vi "Test Indeterminate Progress Bar.vi"() -> ()   [LabVIEW 2020]
panel:
  out "Slide 2":cluster{dbl, dbl}(slide) caption="Running script" scale=0.0..100.0
  out "Slide":cluster{dbl, dbl}(slide) caption="Running script" scale=0.0..100.0
  in  "Stop":bool
  in  "Start":bool
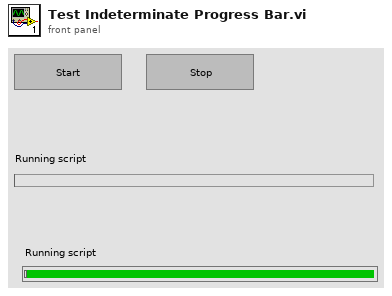
[diagram p1: front panel]
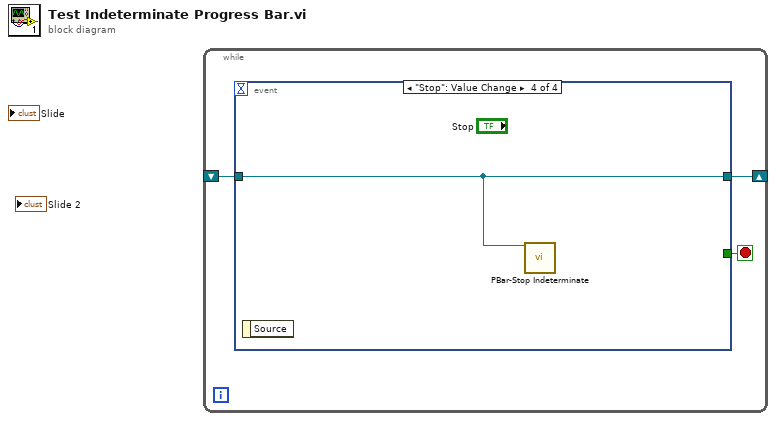
[diagram p0: block diagram]
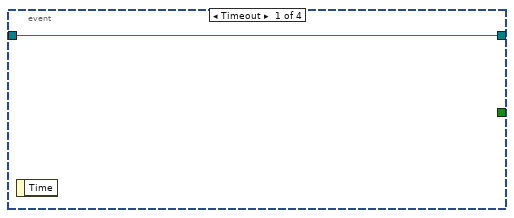
[diagram p2: hidden frame]
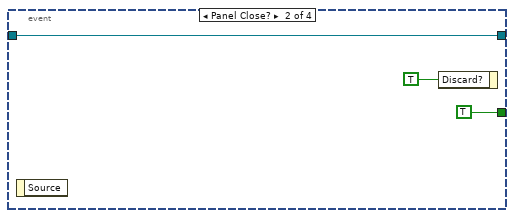
[diagram p3: hidden frame]
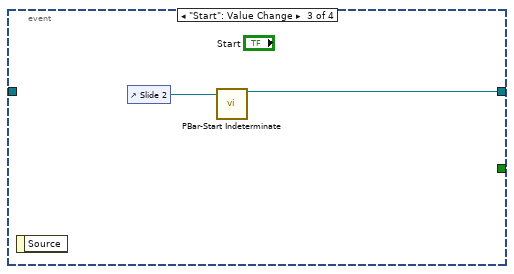
[diagram p4: hidden frame]
diagram:
  n1 = while {
    shift-right: [w2] -> _
    shift-left: _ -> [w1]
    stop <- w3 stop-if-true
    n2 = event shown="[3] \"Stop\": Value Change" {
      selector: _ -> [_ _ _ _]
      dyn-events: _ -> [_ _ _ _]
      timeout: _ -> [_ _ _ _]
      tunnel: [_ TRUE _ _] -> w3
      tunnel: [w4 w5 w8 w10] -> w2
      tunnel: w1 -> [w4 w5 _ w10]
      event Timeout {
        n3 = event-data() -> ()  [unwired: 1 in, 1 out]
      }
      event Panel Close? {
        n4 = event-data() -> ()  [unwired: 1 in, 1 out]
        n5 = event-data("Discard?"=TRUE) -> ()  [unwired: 1 in, 1 out]
      }
      event "Start": Value Change {
        n6 = event-data() -> ()  [unwired: 1 in, 1 out]
        n7 = control-ref of="Slide 2"() -> (w9:refnum<vi>)
        n8 = call "PBar-Start Indeterminate.vi"("Slide"=w9) -> ("reference out"=w8:refnum<vi>)  [unwired: 13 in, 1 out]
      }
      event "Stop": Value Change {
        n9 = event-data() -> ()  [unwired: 1 in, 1 out]
        n10 = call "PBar-Stop Indeterminate.vi"("VI in"=w10) -> ()  [unwired: 14 in, 1 out]
      }
    }
  }
